vi "BNO055 init v.2.vi"(8 "error in (no error)":errorcluster) -> (0 "error out":errorcluster, 3 "I2C out":refnum<class "I2C.lvclass">)   [LabVIEW 2019]
uses:
  FPGA_subVIs/low level/I2C/I2C.lvclass
  <vilib>/myRIO/Instrument Drivers/Onboard IO/I2C/typedefs/I2C User Configuration.ctl
  <vilib>/myRIO/Instrument Drivers/Onboard IO/I2C/typedefs/I2C Transfer Rate.ctl
  <vilib>/myRIO/Instrument Drivers/Onboard IO/I2C/I2C.lvlib
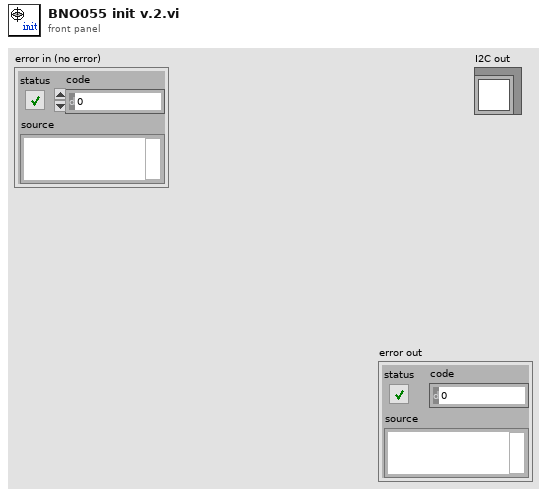
[diagram p1: front panel]
types:
  T1 = typedef "I2C.lvlib/I2C User Configuration.ctl" = cluster{"I2C Transfer Rate":T2}
  T2 = typedef "I2C.lvlib/I2C Transfer Rate.ctl" = enum16{"Standard mode (100 kbps)", "Fast mode (400 kbps)"}
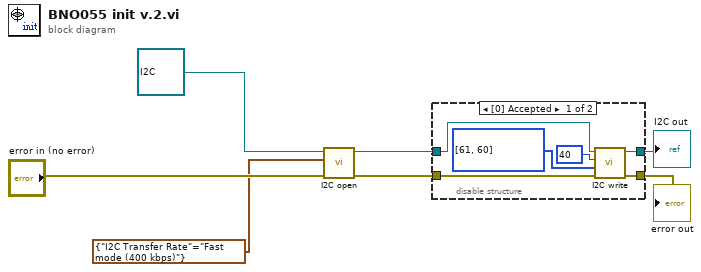
[diagram p0: block diagram]
diagram:
  n1 = call-dynamic "I2C open.vi"("error in (no error)"="error in (no error)", "I2C User Configuration"=T1 {"I2C Transfer Rate"=enum."Fast mode (400 kbps)"}, "I2C in"=refnum<class "I2C.lvclass"> refnum) -> ("error out"=w5:errorcluster, "I2C out"=w2:refnum<class "I2C.lvclass">)  [unwired: 7 in]
  n2 = disable-structure shown="[0] Accepted" {
    disable-tunnel: w2 -> [w13 w15]
    disable-tunnel: [w12 w15] -> w1
    disable-tunnel: w5 -> [w11 w14]
    disable-tunnel: [w10 w14] -> w7
    frame Enabled {
      n3 = call-dynamic "I2C write.vi"("error in (no error)"=w11, "Bytes to Write"=u8[] [61, 60], "Slave Address (7-bit)"=u8 40, "I2C in"=w13) -> ("error out"=w10:errorcluster, "I2C out"=w12:refnum<class "I2C.lvclass">)  [unwired: 6 in]
    }
    frame Disabled {
    }
  }
  "error out" <- w7
  "I2C out" <- w1
